vi "Connection test.vi"() -> ()   [LabVIEW 2021]
uses:
  <vilib>/addons/database/_DB Variant To Data/Database Variant To Data.xnode
  <vilib>/addons/database/Recordset.llb/Rec Destroy - Connection.vi
  <vilib>/addons/database/Connection.llb/Conn Execute.vi
  <vilib>/addons/database/Connection.llb/DB Tools Open Connec (Path).vi
  <vilib>/addons/database/NI_Database_API.lvlib
  <userlib>/LabSQL/LabSQL.lvlib
  <userlib>/sushu/sushu.lvlib
  <vilib>/addons/database/Connection.llb/DB Tools Open Connec (String).vi
panel:
  out "String":string
  out "data":string[][](array[string])
  out "tables":string[](array[string])
  out "error out":errorcluster
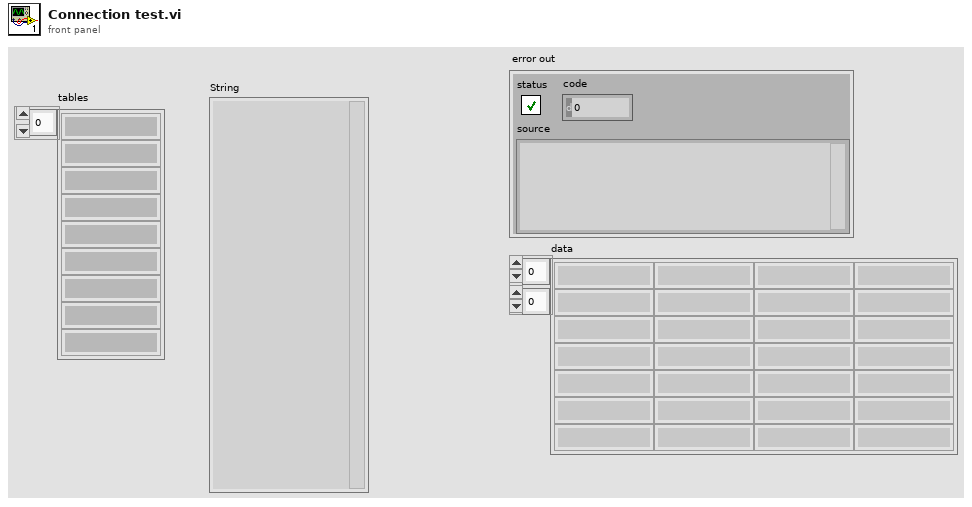
[diagram p1: front panel]
types:
  T1 = typedef "NI_Database_API.lvlib/Conn ObjectReference.ctl" = refnum<k1>
  T2 = enum16{"Other", "SQL2008", "SQLite", "Access", "MySQL"}
  T3 = typedef "NI_Database_API.lvlib/Rec ObjectReference.ctl" = refnum<k1>
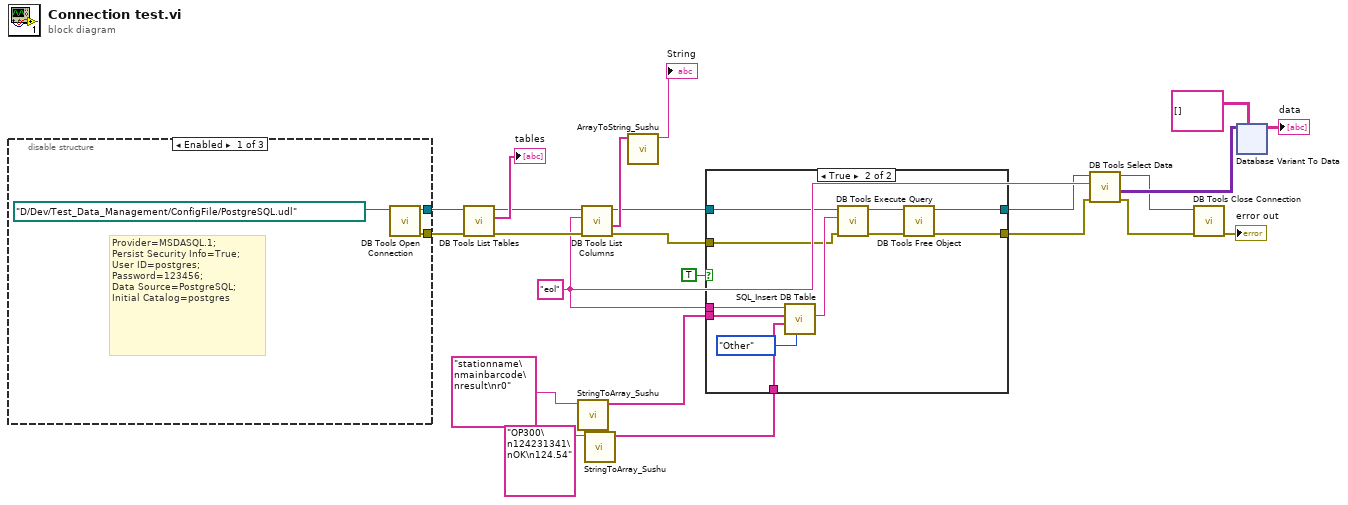
[diagram p0: block diagram]
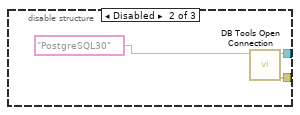
[diagram p3: hidden frame]
diagram:
  w14 = "eol" ("table")
  n1 = disable-structure shown="Enabled" {
    disable-tunnel: [w25 w29 _] -> w22
    disable-tunnel: [w24 w28 _] -> w21
    frame Enabled {
      # "Provider=MSDASQL.1;\nPersist Security Info=True;\nUser ID=postgres;\nPassword=123456;\nData Source=PostgreSQL;\nInitial Catalog=postgres"
      n2 = call-poly <vilib>:"DB Tools Open Connection.vi"("connection information"=path "D:/Dev/Test_Data_Management/ConfigFile/PostgreSQL.udl") -> ("error out"=w24:errorcluster, "connection reference"=w25:T1)  [unwired: 7 in]
    }
    frame Disabled {
      n3 = call-poly <vilib>:"DB Tools Open Connection.vi"("connection information"="PostgreSQL30" ("table")) -> ("error out"=w28:errorcluster, "connection reference"=w29:T1)  [unwired: 7 in]
    }
    frame Disabled {
    }
  }
  n4 = call <vilib>:"DB Tools List Tables.vi"("error in (no error)"=w21, "connection reference"=w22) -> ("error out"=w15:errorcluster, "tables"=→"tables":string[], "connection reference out"=w16:T1)  [unwired: 3 in]
  n5 = call <userlib>:"StringToArray_Sushu.vi"("State Queue"="stationname\nmainbarcode\nresult\nr0") -> ("Array"=w4:string[])  [unwired: 7 in, 3 out]
  n6 = call <vilib>:"DB Tools List Columns.vi"("error in (no error)"=w15, "table"=w14, "connection reference"=w16) -> ("error out"=w11:errorcluster, "columns"=w13:string[], "connection reference out"=w10:T1)  [unwired: 1 in, 1 out]
  n7 = call <userlib>:"StringToArray_Sushu.vi"("State Queue"="OP300\n124231341\nOK\n124.54") -> ("Array"=w3:string[])  [unwired: 7 in, 3 out]
  n8 = call <userlib>:"ArrayToString_Sushu.vi"("Array"=w13) -> ("String"=→"String":string)  [unwired: 10 in]
  n9 = case shown="True" TRUE {
    tunnel: [w31 w40] -> w8
    tunnel: [w30 w39] -> w6
    tunnel: w14 -> [_ w37]
    tunnel: w11 -> [w30 w36]
    tunnel: w10 -> [w31 w35]
    tunnel: w4 -> [_ w34]
    tunnel: w3 -> [_ w33]
    frame False {
    }
    frame True {
      n10 = call <userlib>:"SQL_Insert DB Table.vi"("DB Type"=T2."Other", "ColumnsValue"=w33, "ColumnsName"=w34, "Table Name"=w37) -> ("Insert DB String"=w38:string)  [unwired: 7 in]
      n11 = call-poly <vilib>:"DB Tools Execute Query.vi"("error in (no error)"=w36, "SQL query"=w38, "connection reference"=w35) -> ("error out"=w42:errorcluster, "recordset reference"=w41:T3)  [unwired: 5 in]
      n12 = call-poly <vilib>:"DB Tools Free Object.vi"("error in (no error)"=w42, "recordset reference"=w41) -> ("error out"=w39:errorcluster, "connection reference"=w40:T1)  [unwired: 8 in]
    }
  }
  n13 = call <vilib>:"DB Tools Select Data.vi"("error in (no error)"=w6, "table"=w14, "connection reference"=w8) -> ("error out"=w5:errorcluster, "data"=w19:variant[][], "connection reference out"=w7:T1)  [unwired: 3 in]
  n14 = call <vilib>:"DB Tools Close Connection.vi"("error in (no error)"=w5, "connection reference"=w7) -> ("error out"=→"error out":errorcluster)  [unwired: 5 in]
  n15 = xnode "Database Variant To Data"("database variant"=w19, "type"=string[][] [] ("tables")) -> ("data"=→"data":string[][])  [unwired: 1 in, 1 out]
